vi "FinishFBVarSet.vi"(6 "AccumulatedErrors in":i32, 7 "ExpectedElements":i32, 9 "Finished VarSet":T1, 10 "Command":string, 11 "Queue in":refnum<queue>) -> (0 "queue error out":errorcluster, 1 "Response Data":string, 2 "Response Code":string, 3 "Queue out":refnum<queue>, 4 "AccumulatedErrors out":i32)   [LabVIEW 2013]
uses:
  FBVarSet.ctl
  FBVar.ctl
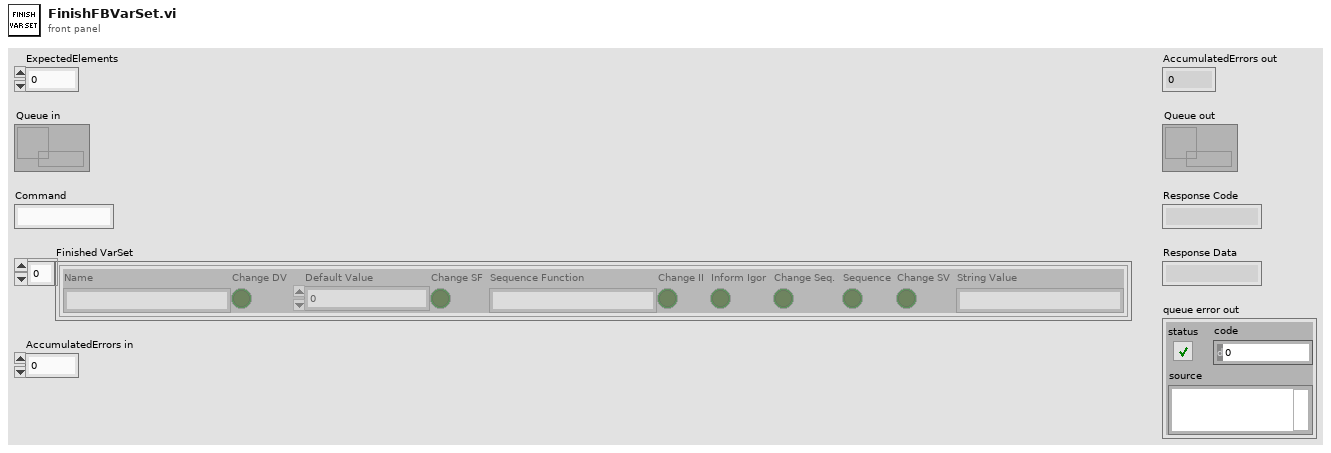
[diagram p1: front panel]
types:
  T1 = typedef "FBVarSet.ctl" = T2[]
  T2 = typedef "FBVar.ctl" = cluster{"Name":string, "Change DV":bool, "Default Value":dbl, "Change SF":bool, "Sequence Function":string, "Change II":bool, "Inform Igor":bool, "Change Seq.":bool, "Sequence":bool, "Change SV":bool, "String Value":string}
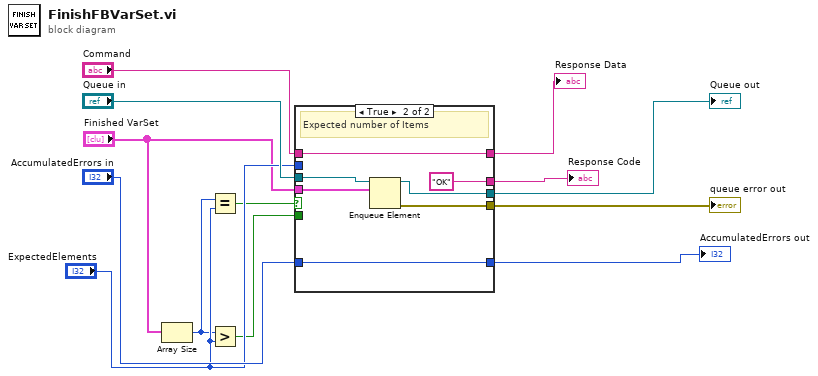
[diagram p0: block diagram]
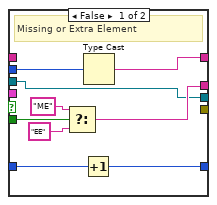
[diagram p2: hidden frame]
diagram:
  n1 = Array Size(array="Finished VarSet") -> (size(s)=w3:i32)
  n2 = Equal?(x=w3, y="ExpectedElements") -> (x = y?=w1:bool)
  n3 = Greater?(x=w3, y="ExpectedElements") -> (0:w4:bool)
  n4 = case shown="True" w1 {
    tunnel: [w16 w29] -> w12
    tunnel: [_ w28] -> w8
    tunnel: [w17 "OK" ("string")] -> w9
    tunnel: "Command" -> [_ w26]
    tunnel: [w18 w26] -> w10
    tunnel: "Queue in" -> [w16 w25]
    tunnel: "Finished VarSet" -> [_ w24]
    tunnel: w4 -> [w20 _]
    tunnel: "ExpectedElements" -> [w19 _]
    tunnel: "AccumulatedErrors in" -> [w15 w23]
    tunnel: [w14 w23] -> w7
    frame False {
      # "Missing or Extra Element"
      n5 = Select(t="ME" ("name (unnamed)"), s=w20, f="EE" ("name (unnamed)")) -> (s? t:f=w17:string)
      n6 = Increment(x=w15) -> (x+1=w14:i32)
      n7 = Type Cast(x=w19) -> (*(type *) &x=w18:string)  [unwired: 1 in]
    }
    frame True {
      # "Expected number of Items"
      n8 = Enqueue Element(queue=w25, element=w24) -> (queue out=w29:refnum<queue>, error out=w28:errorcluster)  [unwired: 2 in, 1 out]
    }
  }
  "Queue out" <- w12
  "Response Data" <- w10
  "Response Code" <- w9
  "queue error out" <- w8
  "AccumulatedErrors out" <- w7
